vi "Driver VISA Initial.vi"(8 "error in":errorcluster, 9 "timeout(ms)":u32=2000, 10 "serial":T1={"baud rate"=9600, "data bits"=8, "parity"=enum."None", "stop bits"=10, "flow control"=0, "Enable Termination\nChar (T)"=TRUE, "termination char\n(0xA = '\\n' = LF) "=10} {"stop bits" items=["1.0"=10, "1.5"=15, "2.0"=20]; "flow control" items=["无", "XON/XOFF", "RTS/CTS", "XON/XOFF & RTS/CTS", "DTR/DSR", "XON/XOFF & DTR/DSR"]}, 11 "visa in":refnum<visa-resource-name>) -> (0 "error out":errorcluster, 3 "visa out":refnum<visa-resource-name>)   [LabVIEW 2020]
uses:
  <vilib>/Instr/_visa.llb/VISA Configure Serial Port (Instr).vi
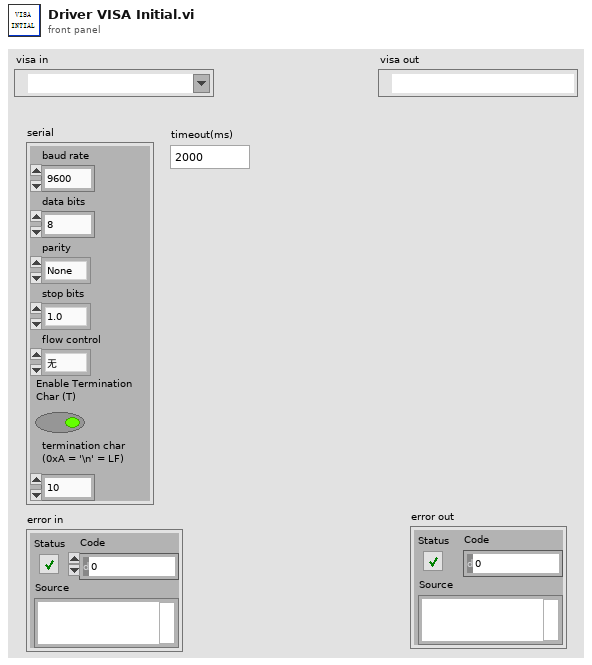
[diagram p1: front panel]
types:
  T1 = cluster{"baud rate":u32, "data bits":u16, "parity":enum16{"None", "Odd", "Even", "Mark", "Space"}, "stop bits":u16, "flow control":u16, "Enable Termination\nChar (T)":bool, "termination char\n(0xA = '\\n' = LF) ":u8}
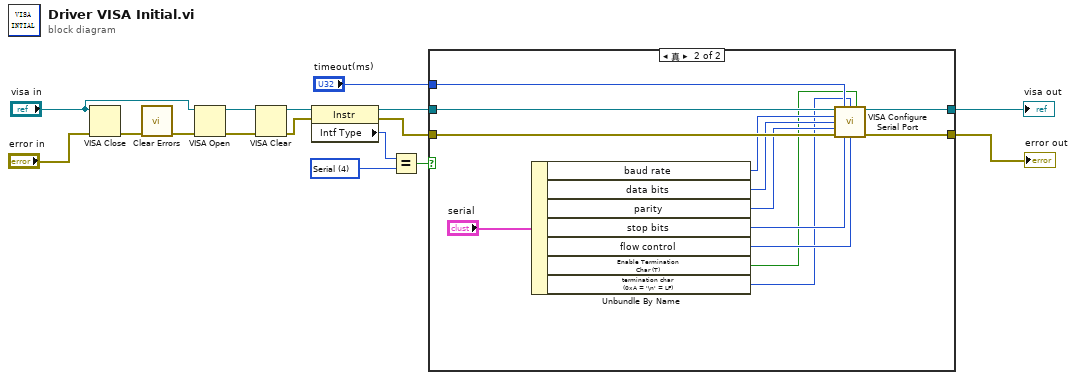
[diagram p0: block diagram]
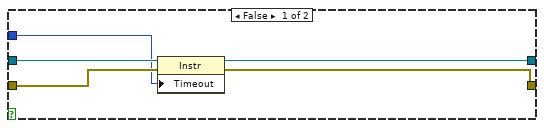
[diagram p2: hidden frame]
diagram:
  w9 = u16 4 items=["GPIB"=1, "VXI"=2, "GPIB-VXI"=3, "Serial"=4, "PXI"=5, "TCPIP"=6, "USB"=7, "FireWire"=9] ("Interface Information:Interface Type")
  n1 = VISA Close(VISA resource name="visa in", error in (no error)="error in") -> (error out=w16:errorcluster)
  n2 = call <vilib>:"Clear Errors.vi"("error in (no error)"=w16) -> ("error out"=w15:errorcluster)  [unwired: 5 in, 1 out]
  n3 = VISA Open(error in (no error)=w15, VISA resource name="visa in") -> (VISA resource name=w13:refnum<visa-resource-name>, error out=w14:errorcluster)  [unwired: 3 in]
  n4 = VISA Clear(VISA resource name=w13, error in (no error)=w14) -> (VISA resource name out=w12:refnum<visa-resource-name>, error out=w11:errorcluster)
  n5 = property class="Instr"(reference=w12, error in=w11) -> (reference out=w7:refnum<visa-resource-name>, error out=w6:errorcluster, "Intf Type"=w10:u16)
  n6 = Equal?(x=w10, y=w9) -> (x = y?=w8:bool)
  n7 = case shown="真" w8 {
    tunnel: w7 -> [w21 w34]
    tunnel: w6 -> [w20 w33]
    tunnel: [w19 w31] -> w3
    tunnel: [w18 w30] -> w2
    tunnel: "timeout(ms)" -> [w17 w32]
    frame False {
      n8 = property class="Instr"(reference=w21, error in=w20, "Timeout"=w17) -> (reference out=w19:refnum<visa-resource-name>, error out=w18:errorcluster)
    }
    frame True {
      n9 = Unbundle By Name("serial") -> ("baud rate"=w28:u32, "data bits"=w27:u16, "parity"=w26:enum16{"None", "Odd", "Even", "Mark", "Space"}, "stop bits"=w25:u16, "flow control"=w24:u16, "Enable Termination\nChar (T)"=w23:bool, "termination char\n(0xA = '\\n' = LF)"=w22:u8)
      n10 = call-poly "VISA Configure Serial Port"("VISA resource name"=w34, "timeout (10sec)"=w32, "termination char\n(0xA = '\\n' = LF)"=w22, "Enable Termination\nChar (T)"=w23, "baud rate (9600)"=w28, "data bits (8)"=w27, "parity (0:none)"=w26, "error in (no error)"=w33, "stop bits (10: 1 bit)"=w25, "flow control (0:none)"=w24) -> ("VISA resource name out"=w31:refnum<visa-resource-name>, "error out"=w30:errorcluster)  [unwired: 4 in]
    }
  }
  "error out" <- w2
  "visa out" <- w3
